vi "config_ini.vi"(9 "no article":string) -> (0 "subarray":variant[](array[variant]))   [LabVIEW 2014]
uses:
  <vilib>/addons/database/Connection.llb/DB Tools Open Connec (String).vi
  <vilib>/addons/database/Connection.llb/Conn Execute.vi
  <vilib>/addons/database/Recordset.llb/Rec Fetch Recordset Data (R).vi
  <vilib>/addons/database/Recordset.llb/Rec Destroy - Connection.vi
  FT_HMI.llb/GLOBAL_PUMPS_PARAMS.vi
  <vilib>/addons/database/NI_Database_API.lvlib
panel:
  out "no article 3":string
  out "no article 2":string
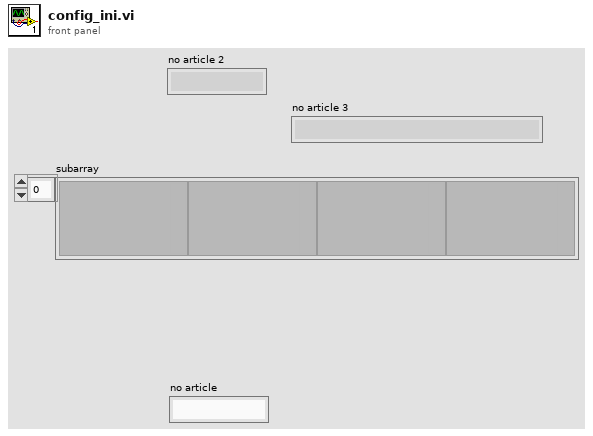
[diagram p1: front panel]
types:
  T1 = typedef "NI_Database_API.lvlib/Conn ObjectReference.ctl" = refnum<k1>
  T2 = typedef "NI_Database_API.lvlib/Rec ObjectReference.ctl" = refnum<k1>
  T3 = cluster{"GENERAL":cluster{"NO ARTICLE":string, "DESIGNATION":string, "TENSION [V]":sgl, "FREQUENCE [Hz]":sgl, "BYPASS":bool}, "ST1_HT":cluster{"STATUS HT":bool, "TENSION ISOLATION [V]":sgl, "COURANT ISOLATION [mA]":sgl, "TEMPS DE MESURE [ms]":i32, "NO PROGRAMME":i32}, "ST2_ASPIRATION":cluster{"STATUS H ASP":bool, "TEMPS POMPAGE [ms]":i32, "STATUS CONTRE-PRESSION":bool, "HAUTEUR ASPIRATION [m]":sgl, "TEMPS DE MESURE ASP [ms]":i32, "STATUS PERTE ASP":bool, "PERTE ASPIRATION [mbar]":sgl, "TEMPS DE MESURE PERTE [ms] ":i32}, "ST3_ETANCHEITE":cluster{"STATUS":bool, "ETANCHEITE [mbar]":sgl, "TEMPS MISE SOUS PRESSION [ms]":i32, "TEMPS STABILISATION [ms]":i32, "TEMPS DE MESURE [ms]":i32}, "ST4-5_DEBIT":cluster{"STATUS QMAX":bool, "GRAND DEBIT":bool, "PUMPING_TIME  [ms]":i32, "DEBIT MIN [l/h]":sgl, "DEBIT MAX  [l/h]":sgl, "TEMPS DE MESURE QMAX [ms]":i32, "STATUS QTRAVAIL 1":bool, "DEBIT TRAVAIL 1 MIN [l/h]":sgl, "DEBIT TRAVAIL 1 MAX [l/h]":sgl, "PRESSION DE CONSIGNE 1 [bar]":sgl, "TEMPS DE REGLAGE PRESSION [ms]":i32, "TEMPS DE MESURE QTRAVAIL 1 [ms]":i32, "STATUS QTRAVAIL 2":bool, "DEBIT TRAVAIL 2 MIN [l/h]":sgl, "DEBIT TRAVAIL 2 MAX [l/h]":sgl, "PRESSION DE CONSIGNE 2 [bar]":sgl, "TEMPS DE MESURE QTRAVAIL 2 [ms]":i32, "STATUS CONSO":bool, "CONSOMMATION [A]":sgl, "TEMPS DE MESURE COURANT [ms]":i32}, "ST6_PRESSION":cluster{"STATUS PMAX":bool, "PUMPING TIME [ms]":i32, "PRESSION MIN [bar]":sgl, "TEMPS DE MESURE PMAX [ms]":i32, "STATUS PERTE PRESSION":bool, "PERTE PRESSION [mbar]":sgl, "TEMPS DE MESURE PERTE [ms]":i32}, "ST7_VIDANGE":cluster{"STATUS VIDANGE":bool, "TEMPS DE VIDANGE [ms] ":i32}, "ST8_IMPRESSION":cluster{"STATUS":bool, "ETIQUETTE":string}, "ST9_DECHARGEMENT":cluster{"STATUS":bool, "BOBINE A FIL":bool}, "DIVERS":cluster{"INDICE MODIF":string, "DATE MODIF":timestamp, "HISTORIQUE MODIF":string, "EMBOUT PRESSION":string, "EMBOUT ASPIRATION":string}}
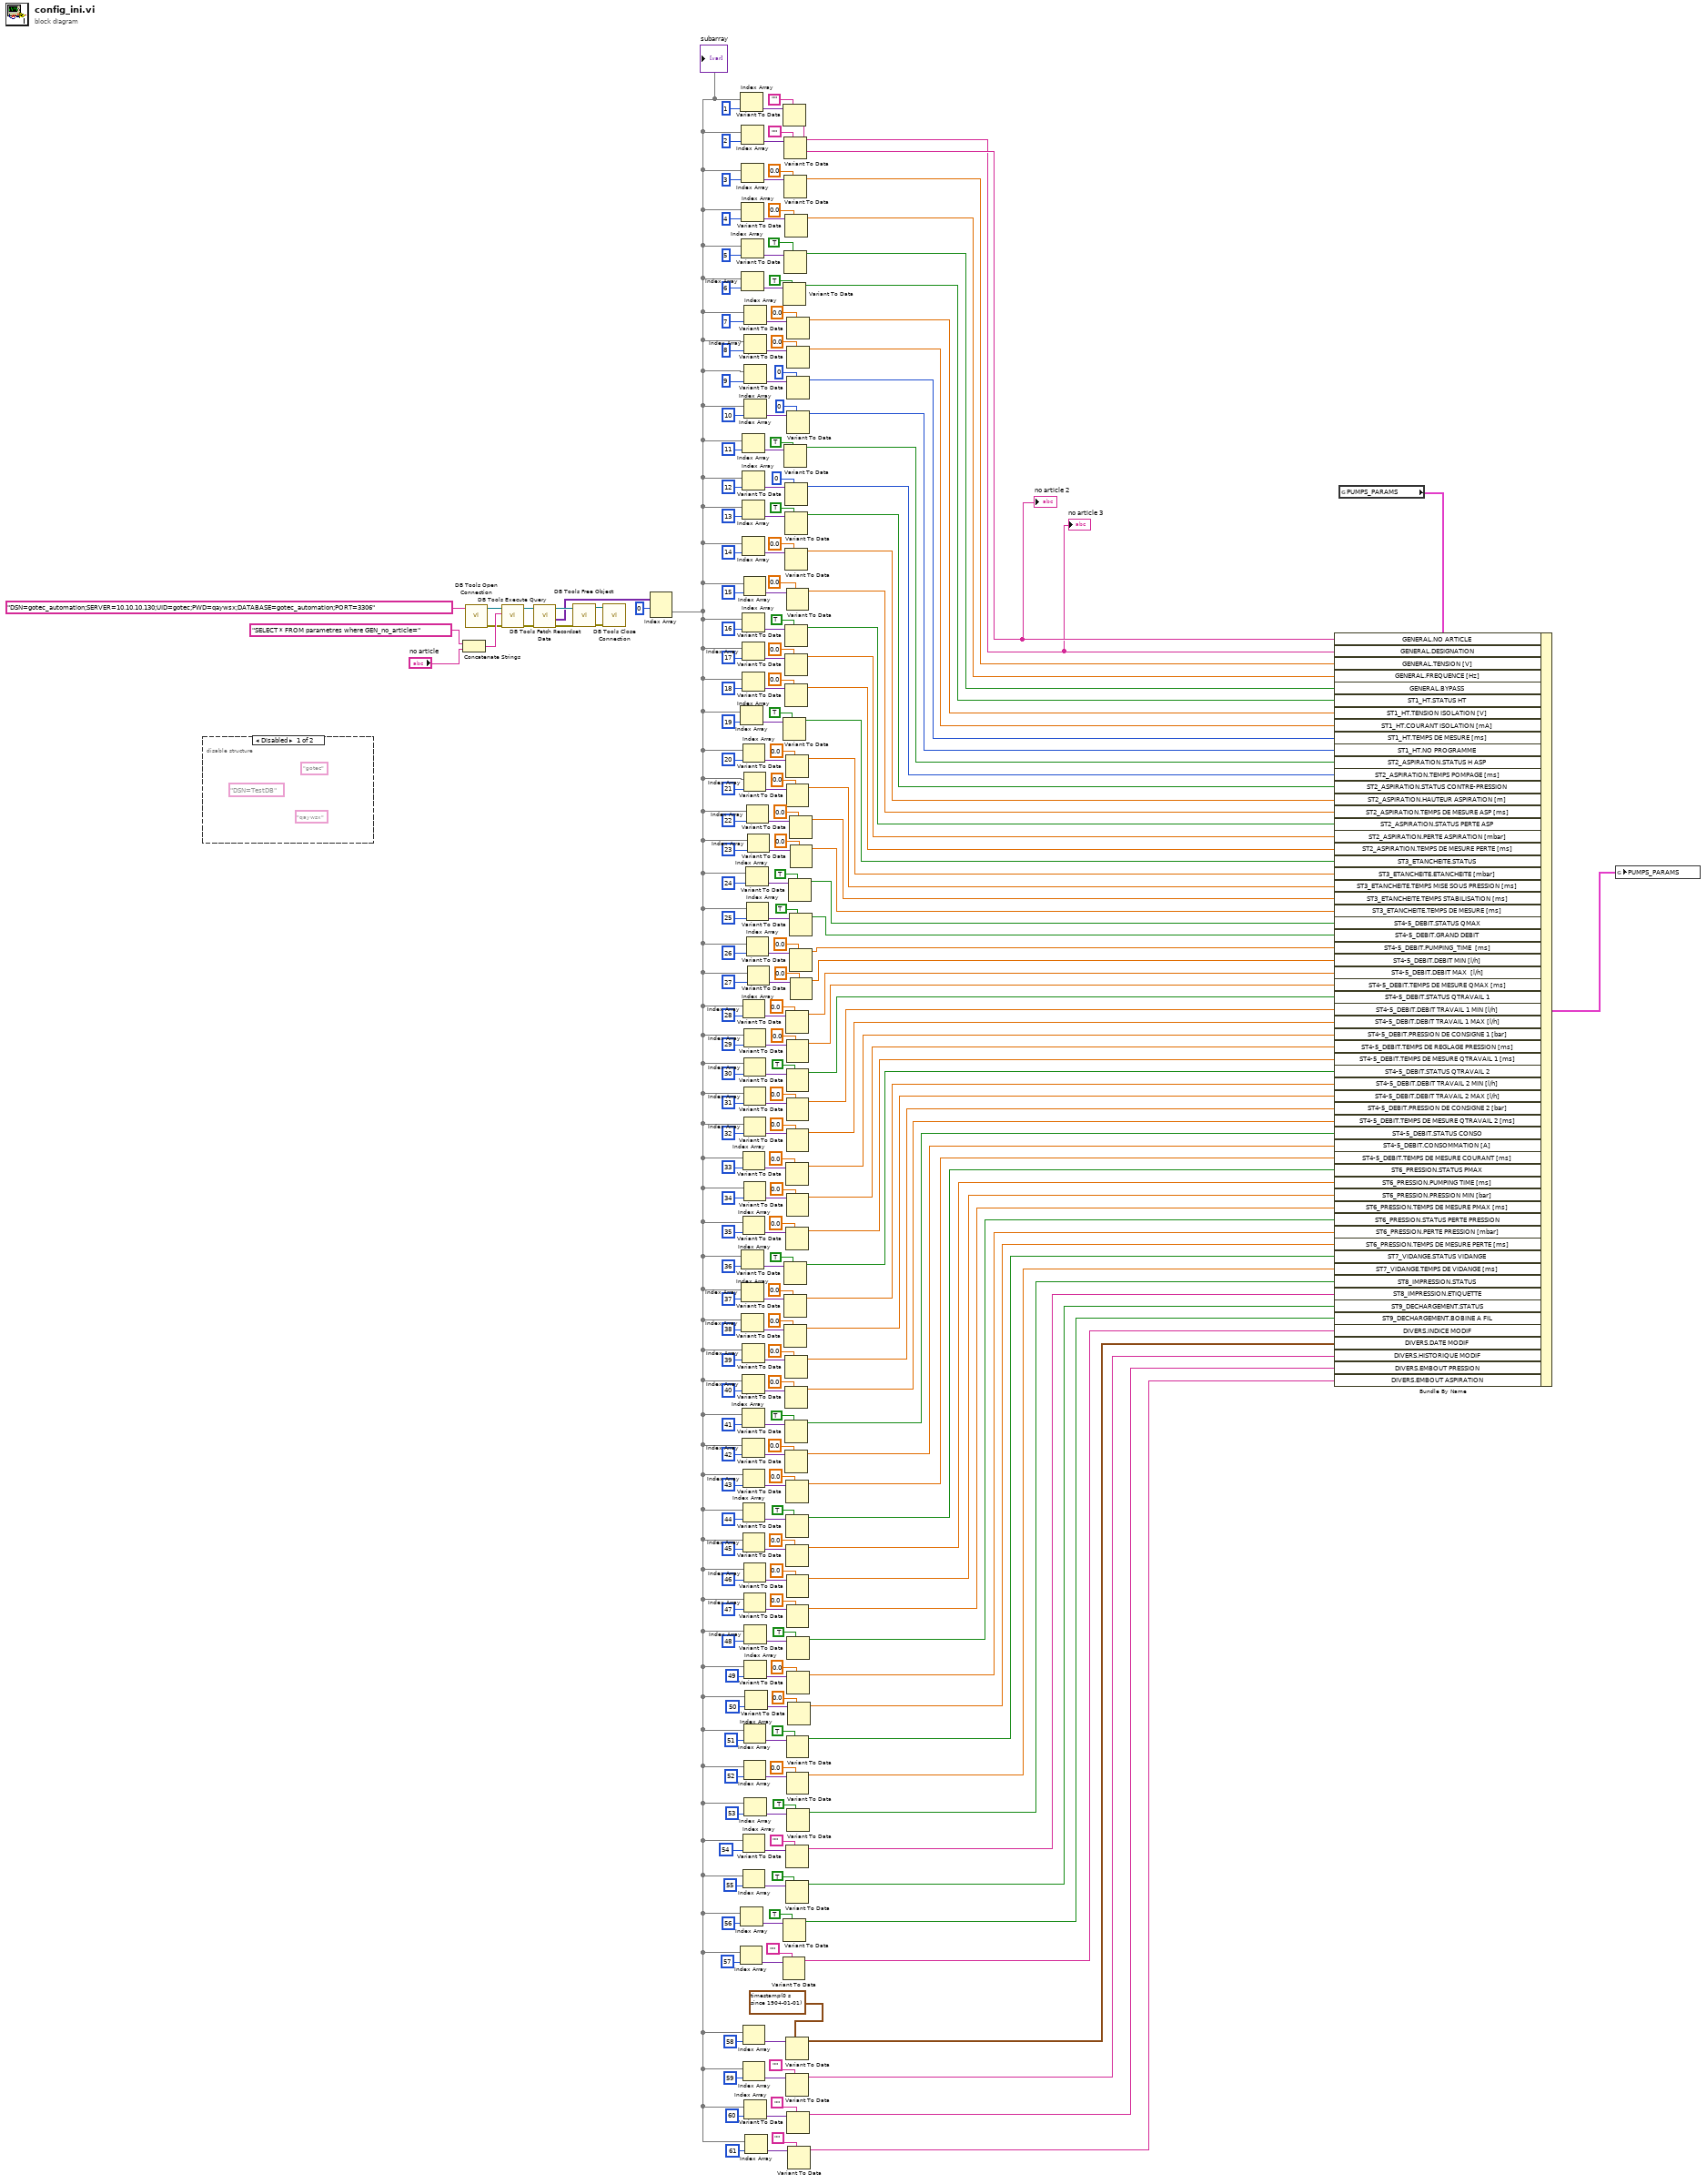
[diagram p0: block diagram]
diagram:
  n1 = disable-structure shown="Disabled" {
    frame Disabled {
      (unwired) "qaywsx" ("password")
      (unwired) "gotec" ("userID")
      (unwired) "DSN=TestDB"
    }
    frame Enabled {
    }
  }
  n2 = Concatenate Strings("SELECT * FROM parametres where GEN_no_article=" ("SQL query"), "no article") -> (w256:string)
  n3 = call-poly <vilib>:"DB Tools Open Connection.vi"("connection information"="DSN=gotec_automation;SERVER=10.10.10.130;UID=gotec;PWD=qaywsx;DATABASE=gotec_automation;PORT=3306") -> ("error out"=w253:errorcluster, "connection reference"=w254:T1)  [unwired: 7 in]
  n4 = call-poly <vilib>:"DB Tools Execute Query.vi"("error in (no error)"=w253, "SQL query"=w256, "connection reference"=w254) -> ("error out"=w258:errorcluster, "recordset reference"=w260:T2)  [unwired: 5 in]
  n5 = call-poly <vilib>:"DB Tools Fetch Recordset Data.vi"("error in (no error)"=w258, "recordset reference"=w260) -> ("error out"=w257:errorcluster, "recordset data"=w134:variant[][], "recordset reference out"=w259:T2)  [unwired: 3 in]
  n6 = call-poly <vilib>:"DB Tools Free Object.vi"("error in (no error)"=w257, "recordset reference"=w259) -> ("error out"=w261:errorcluster, "connection reference"=w251:T1)  [unwired: 8 in]
  n7 = call <vilib>:"DB Tools Close Connection.vi"("error in (no error)"=w261, "connection reference"=w251) -> ()  [unwired: 5 in, 1 out]
  n8 = Index Array(array=w134, index (row)=0 ("index")) -> (element=w5:variant[])  [unwired: 1 in]
  "subarray" <- w5
  n9 = Index Array(array=w5, index=57) -> (element=w141:variant)
  n10 = Index Array(array=w5, index=1) -> (element=w196:variant)
  n11 = Index Array(array=w5, index=19) -> (element=w193:variant)
  n12 = Index Array(array=w5, index=56) -> (element=w144:variant)
  n13 = Index Array(array=w5, index=2) -> (element=w199:variant)
  n14 = Index Array(array=w5, index=3) -> (element=w250:variant)
  n15 = Index Array(array=w5, index=4) -> (element=w247:variant)
  n16 = Index Array(array=w5, index=5) -> (element=w132:variant)
  n17 = Index Array(array=w5, index=6) -> (element=w121:variant)
  n18 = Index Array(array=w5, index=36) -> (element=w189:variant)
  n19 = Index Array(array=w5, index=37) -> (element=w186:variant)
  n20 = Index Array(array=w5, index=38) -> (element=w183:variant)
  n21 = Index Array(array=w5, index=11) -> (element=w241:variant)
  n22 = Index Array(array=w5, index=12) -> (element=w239:variant)
  n23 = Index Array(array=w5, index=13) -> (element=w236:variant)
  n24 = Index Array(array=w5, index=14) -> (element=w234:variant)
  n25 = Index Array(array=w5, index=16) -> (element=w225:variant)
  n26 = Index Array(array=w5, index=17) -> (element=w222:variant)
  n27 = Index Array(array=w5, index=18) -> (element=w219:variant)
  n28 = Index Array(array=w5, index=39) -> (element=w180:variant)
  n29 = Index Array(array=w5, index=40) -> (element=w177:variant)
  n30 = Index Array(array=w5, index=41) -> (element=w174:variant)
  n31 = Index Array(array=w5, index=42) -> (element=w171:variant)
  n32 = Index Array(array=w5, index=20) -> (element=w106:variant)
  n33 = Index Array(array=w5, index=28) -> (element=w216:variant)
  n34 = Index Array(array=w5, index=33) -> (element=w68:variant)
  n35 = Index Array(array=w5, index=35) -> (element=w59:variant)
  n36 = Index Array(array=w5, index=43) -> (element=w168:variant)
  n37 = Index Array(array=w5, index=44) -> (element=w165:variant)
  n38 = Index Array(array=w5, index=45) -> (element=w162:variant)
  n39 = Index Array(array=w5, index=54) -> (element=w33:variant)
  n40 = Index Array(array=w5, index=55) -> (element=w25:variant)
  n41 = Index Array(array=w5, index=58) -> (element=w16:variant)
  n42 = Index Array(array=w5, index=59) -> (element=w19:variant)
  n43 = Index Array(array=w5, index=15) -> (element=w228:variant)
  n44 = Index Array(array=w5, index=21) -> (element=w103:variant)
  n45 = Index Array(array=w5, index=29) -> (element=w210:variant)
  n46 = Index Array(array=w5, index=30) -> (element=w207:variant)
  n47 = Index Array(array=w5, index=31) -> (element=w205:variant)
  n48 = Index Array(array=w5, index=32) -> (element=w202:variant)
  n49 = Index Array(array=w5, index=34) -> (element=w65:variant)
  n50 = Index Array(array=w5, index=46) -> (element=w159:variant)
  n51 = Index Array(array=w5, index=47) -> (element=w48:variant)
  n52 = Index Array(array=w5, index=51) -> (element=w38:variant)
  n53 = Index Array(array=w5, index=52) -> (element=w147:variant)
  n54 = Index Array(array=w5, index=7) -> (element=w119:variant)
  n55 = Index Array(array=w5, index=8) -> (element=w118:variant)
  n56 = Index Array(array=w5, index=9) -> (element=w117:variant)
  n57 = Index Array(array=w5, index=10) -> (element=w116:variant)
  n58 = Index Array(array=w5, index=48) -> (element=w156:variant)
  n59 = Index Array(array=w5, index=49) -> (element=w153:variant)
  n60 = Index Array(array=w5, index=53) -> (element=w30:variant)
  n61 = Index Array(array=w5, index=60) -> (element=w11:variant)
  n62 = Index Array(array=w5, index=50) -> (element=w150:variant)
  n63 = Index Array(array=w5, index=61) -> (element=w8:variant)
  n64 = Index Array(array=w5, index=24) -> (element=w90:variant)
  n65 = Index Array(array=w5, index=22) -> (element=w100:variant)
  n66 = Index Array(array=w5, index=25) -> (element=w87:variant)
  n67 = Index Array(array=w5, index=26) -> (element=w82:variant)
  n68 = Index Array(array=w5, index=23) -> (element=w97:variant)
  n69 = Index Array(array=w5, index=27) -> (element=w79:variant)
  n70 = Variant To Data(type="", Variant=w141) -> (data=w14:string)  [unwired: 1 in, 1 out]
  n71 = Variant To Data(type="", Variant=w196) -> (data=w139:string)  [unwired: 1 in, 1 out]
  "no article 2" <- w139
  n72 = Variant To Data(type=TRUE, Variant=w121) -> (data=w120:bool)  [unwired: 1 in, 1 out]
  n73 = Variant To Data(type=TRUE, Variant=w193) -> (data=w190:bool)  [unwired: 1 in, 1 out]
  n74 = Variant To Data(type=TRUE, Variant=w144) -> (data=w21:bool)  [unwired: 1 in, 1 out]
  n75 = Variant To Data(type="", Variant=w199) -> (data=w138:string)  [unwired: 1 in, 1 out]
  "no article 3" <- w138
  n76 = Variant To Data(type=sgl 0.0, Variant=w250) -> (data=w133:sgl)  [unwired: 1 in, 1 out]
  n77 = Variant To Data(type=TRUE, Variant=w132) -> (data=w130:bool)  [unwired: 1 in, 1 out]
  n78 = Variant To Data(type=TRUE, Variant=w241) -> (data=w109:bool)  [unwired: 1 in, 1 out]
  n79 = Variant To Data(type=TRUE, Variant=w189) -> (data=w60:bool)  [unwired: 1 in, 1 out]
  n80 = Variant To Data(type=sgl 0.0, Variant=w186) -> (data=w55:sgl)  [unwired: 1 in, 1 out]
  n81 = Variant To Data(type=sgl 0.0, Variant=w183) -> (data=w54:sgl)  [unwired: 1 in, 1 out]
  n82 = Variant To Data(type=sgl 0.0, Variant=w247) -> (data=w135:sgl)  [unwired: 1 in, 1 out]
  n83 = Variant To Data(type=0, Variant=w239) -> (data=w231:i32)  [unwired: 1 in, 1 out]
  n84 = Variant To Data(type=TRUE, Variant=w236) -> (data=w230:bool)  [unwired: 1 in, 1 out]
  n85 = Variant To Data(type=sgl 0.0, Variant=w234) -> (data=w229:sgl)  [unwired: 1 in, 1 out]
  n86 = Variant To Data(type=TRUE, Variant=w225) -> (data=w213:bool)  [unwired: 1 in, 1 out]
  n87 = Variant To Data(type=sgl 0.0, Variant=w222) -> (data=w212:sgl)  [unwired: 1 in, 1 out]
  n88 = Variant To Data(type=sgl 0.0, Variant=w219) -> (data=w211:sgl)  [unwired: 1 in, 1 out]
  n89 = Variant To Data(type=sgl 0.0, Variant=w180) -> (data=w53:sgl)  [unwired: 1 in, 1 out]
  n90 = Variant To Data(type=sgl 0.0, Variant=w177) -> (data=w52:sgl)  [unwired: 1 in, 1 out]
  n91 = Variant To Data(type=TRUE, Variant=w174) -> (data=w51:bool)  [unwired: 1 in, 1 out]
  n92 = Variant To Data(type=sgl 0.0, Variant=w171) -> (data=w50:sgl)  [unwired: 1 in, 1 out]
  n93 = Variant To Data(type=sgl 0.0, Variant=w106) -> (data=w94:sgl)  [unwired: 1 in, 1 out]
  n94 = Variant To Data(type=sgl 0.0, Variant=w216) -> (data=w73:sgl)  [unwired: 1 in, 1 out]
  n95 = Variant To Data(type=sgl 0.0, Variant=w68) -> (data=w62:sgl)  [unwired: 1 in, 1 out]
  n96 = Variant To Data(type=sgl 0.0, Variant=w59) -> (data=w56:sgl)  [unwired: 1 in, 1 out]
  n97 = Variant To Data(type=sgl 0.0, Variant=w168) -> (data=w49:sgl)  [unwired: 1 in, 1 out]
  n98 = Variant To Data(type=TRUE, Variant=w165) -> (data=w46:bool)  [unwired: 1 in, 1 out]
  n99 = Variant To Data(type=sgl 0.0, Variant=w162) -> (data=w45:sgl)  [unwired: 1 in, 1 out]
  n100 = Variant To Data(type="", Variant=w33) -> (data=w26:string)  [unwired: 1 in, 1 out]
  n101 = Variant To Data(type=TRUE, Variant=w25) -> (data=w22:bool)  [unwired: 1 in, 1 out]
  n102 = Variant To Data(type=timestamp(0 s since 1904-01-01) ("DIVERS.DATE MODIF"), Variant=w16) -> (data=w12:timestamp)  [unwired: 1 in, 1 out]
  n103 = Variant To Data(type="", Variant=w19) -> (data=w4:string)  [unwired: 1 in, 1 out]
  n104 = Variant To Data(type=sgl 0.0, Variant=w228) -> (data=w226:sgl)  [unwired: 1 in, 1 out]
  n105 = Variant To Data(type=sgl 0.0, Variant=w103) -> (data=w93:sgl)  [unwired: 1 in, 1 out]
  n106 = Variant To Data(type=sgl 0.0, Variant=w210) -> (data=w72:sgl)  [unwired: 1 in, 1 out]
  n107 = Variant To Data(type=TRUE, Variant=w207) -> (data=w71:bool)  [unwired: 1 in, 1 out]
  n108 = Variant To Data(type=sgl 0.0, Variant=w205) -> (data=w70:sgl)  [unwired: 1 in, 1 out]
  n109 = Variant To Data(type=sgl 0.0, Variant=w202) -> (data=w69:sgl)  [unwired: 1 in, 1 out]
  n110 = Variant To Data(type=sgl 0.0, Variant=w65) -> (data=w61:sgl)  [unwired: 1 in, 1 out]
  n111 = Variant To Data(type=sgl 0.0, Variant=w159) -> (data=w44:sgl)  [unwired: 1 in, 1 out]
  n112 = Variant To Data(type=sgl 0.0, Variant=w48) -> (data=w42:sgl)  [unwired: 1 in, 1 out]
  n113 = Variant To Data(type=TRUE, Variant=w38) -> (data=w35:bool)  [unwired: 1 in, 1 out]
  n114 = Variant To Data(type=sgl 0.0, Variant=w147) -> (data=w34:sgl)  [unwired: 1 in, 1 out]
  n115 = Variant To Data(type=sgl 0.0, Variant=w119) -> (data=w112:sgl)  [unwired: 1 in, 1 out]
  n116 = Variant To Data(type=sgl 0.0, Variant=w118) -> (data=w111:sgl)  [unwired: 1 in, 1 out]
  n117 = Variant To Data(type=0, Variant=w117) -> (data=w110:i32)  [unwired: 1 in, 1 out]
  n118 = Variant To Data(type=0, Variant=w116) -> (data=w113:i32)  [unwired: 1 in, 1 out]
  n119 = Variant To Data(type=TRUE, Variant=w156) -> (data=w41:bool)  [unwired: 1 in, 1 out]
  n120 = Variant To Data(type=sgl 0.0, Variant=w153) -> (data=w40:sgl)  [unwired: 1 in, 1 out]
  n121 = Variant To Data(type=TRUE, Variant=w30) -> (data=w27:bool)  [unwired: 1 in, 1 out]
  n122 = Variant To Data(type="", Variant=w11) -> (data=w3:string)  [unwired: 1 in, 1 out]
  n123 = Variant To Data(type=sgl 0.0, Variant=w150) -> (data=w39:sgl)  [unwired: 1 in, 1 out]
  n124 = Variant To Data(type="", Variant=w8) -> (data=w2:string)  [unwired: 1 in, 1 out]
  n125 = Variant To Data(type=TRUE, Variant=w90) -> (data=w84:bool)  [unwired: 1 in, 1 out]
  n126 = Variant To Data(type=sgl 0.0, Variant=w100) -> (data=w92:sgl)  [unwired: 1 in, 1 out]
  n127 = Variant To Data(type=TRUE, Variant=w87) -> (data=w83:bool)  [unwired: 1 in, 1 out]
  n128 = Variant To Data(type=sgl 0.0, Variant=w82) -> (data=w75:sgl)  [unwired: 1 in, 1 out]
  n129 = Variant To Data(type=sgl 0.0, Variant=w97) -> (data=w91:sgl)  [unwired: 1 in, 1 out]
  n130 = Variant To Data(type=sgl 0.0, Variant=w79) -> (data=w74:sgl)  [unwired: 1 in, 1 out]
  n131 = global read "GLOBAL_PUMPS_PARAMS.vi" "PUMPS_PARAMS"() -> (w243:T3)
  n132 = Bundle By Name(cluster=w243, "GENERAL.NO ARTICLE"=w139, "GENERAL.DESIGNATION"=w138, "GENERAL.TENSION [V]"=w133, "GENERAL.FREQUENCE [Hz]"=w135, "GENERAL.BYPASS"=w130, "ST1_HT.STATUS HT"=w120, "ST1_HT.TENSION ISOLATION [V]"=w112, "ST1_HT.COURANT ISOLATION [mA]"=w111, "ST1_HT.TEMPS DE MESURE [ms]"=w110, "ST1_HT.NO PROGRAMME"=w113, "ST2_ASPIRATION.STATUS H ASP"=w109, "ST2_ASPIRATION.TEMPS POMPAGE [ms]"=w231, "ST2_ASPIRATION.STATUS CONTRE-PRESSION"=w230, "ST2_ASPIRATION.HAUTEUR ASPIRATION [m]"=w229, "ST2_ASPIRATION.TEMPS DE MESURE ASP [ms]"=w226, "ST2_ASPIRATION.STATUS PERTE ASP"=w213, "ST2_ASPIRATION.PERTE ASPIRATION [mbar]"=w212, "ST2_ASPIRATION.TEMPS DE MESURE PERTE [ms]"=w211, "ST3_ETANCHEITE.STATUS"=w190, "ST3_ETANCHEITE.ETANCHEITE [mbar]"=w94, "ST3_ETANCHEITE.TEMPS MISE SOUS PRESSION [ms]"=w93, "ST3_ETANCHEITE.TEMPS STABILISATION [ms]"=w92, "ST3_ETANCHEITE.TEMPS DE MESURE [ms]"=w91, "ST4-5_DEBIT.STATUS QMAX"=w84, "ST4-5_DEBIT.GRAND DEBIT"=w83, "ST4-5_DEBIT.PUMPING_TIME  [ms]"=w75, "ST4-5_DEBIT.DEBIT MIN [l/h]"=w74, "ST4-5_DEBIT.DEBIT MAX  [l/h]"=w73, "ST4-5_DEBIT.TEMPS DE MESURE QMAX [ms]"=w72, "ST4-5_DEBIT.STATUS QTRAVAIL 1"=w71, "ST4-5_DEBIT.DEBIT TRAVAIL 1 MIN [l/h]"=w70, "ST4-5_DEBIT.DEBIT TRAVAIL 1 MAX [l/h]"=w69, "ST4-5_DEBIT.PRESSION DE CONSIGNE 1 [bar]"=w62, "ST4-5_DEBIT.TEMPS DE REGLAGE PRESSION [ms]"=w61, "ST4-5_DEBIT.TEMPS DE MESURE QTRAVAIL 1 [ms]"=w56, "ST4-5_DEBIT.STATUS QTRAVAIL 2"=w60, "ST4-5_DEBIT.DEBIT TRAVAIL 2 MIN [l/h]"=w55, "ST4-5_DEBIT.DEBIT TRAVAIL 2 MAX [l/h]"=w54, "ST4-5_DEBIT.PRESSION DE CONSIGNE 2 [bar]"=w53, "ST4-5_DEBIT.TEMPS DE MESURE QTRAVAIL 2 [ms]"=w52, "ST4-5_DEBIT.STATUS CONSO"=w51, "ST4-5_DEBIT.CONSOMMATION [A]"=w50, "ST4-5_DEBIT.TEMPS DE MESURE COURANT [ms]"=w49, "ST6_PRESSION.STATUS PMAX"=w46, "ST6_PRESSION.PUMPING TIME [ms]"=w45, "ST6_PRESSION.PRESSION MIN [bar]"=w44, "ST6_PRESSION.TEMPS DE MESURE PMAX [ms]"=w42, "ST6_PRESSION.STATUS PERTE PRESSION"=w41, "ST6_PRESSION.PERTE PRESSION [mbar]"=w40, "ST6_PRESSION.TEMPS DE MESURE PERTE [ms]"=w39, "ST7_VIDANGE.STATUS VIDANGE"=w35, "ST7_VIDANGE.TEMPS DE VIDANGE [ms]"=w34, "ST8_IMPRESSION.STATUS"=w27, "ST8_IMPRESSION.ETIQUETTE"=w26, "ST9_DECHARGEMENT.STATUS"=w22, "ST9_DECHARGEMENT.BOBINE A FIL"=w21, "DIVERS.INDICE MODIF"=w14, "DIVERS.DATE MODIF"=w12, "DIVERS.HISTORIQUE MODIF"=w4, "DIVERS.EMBOUT PRESSION"=w3, "DIVERS.EMBOUT ASPIRATION"=w2) -> (w244:T3)
  n133 = global write "GLOBAL_PUMPS_PARAMS.vi" "PUMPS_PARAMS"(w244) -> ()
